vi "#241_MAV_MSG_VIBRATION_DECODE.vi"(11 "mavlink_payload":u8[](array[numeric])) -> (3 "VIBRATION":T1)   [LabVIEW 2023]
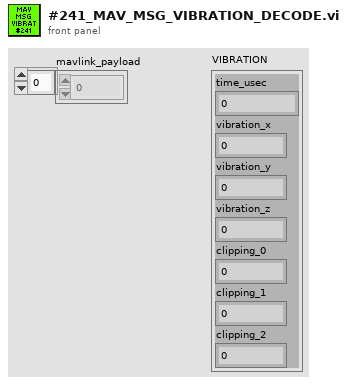
[diagram p1: front panel]
types:
  T1 = cluster{"time_usec":u64, "vibration_x":sgl, "vibration_y":sgl, "vibration_z":sgl, "clipping_0":u32, "clipping_1":u32, "clipping_2":u32}
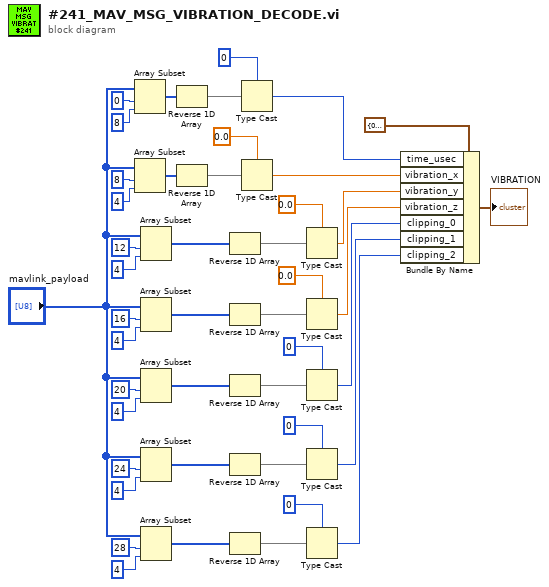
[diagram p0: block diagram]
diagram:
  n1 = Array Subset(array="mavlink_payload", index=0 ("Index"), length=8) -> (w42:u8[])
  n2 = Array Subset(array="mavlink_payload", index=8 ("Index"), length=4) -> (w36:u8[])
  n3 = Array Subset(array="mavlink_payload", index=12 ("Index"), length=4) -> (w30:u8[])
  n4 = Array Subset(array="mavlink_payload", index=16 ("Index"), length=4) -> (w24:u8[])
  n5 = Array Subset(array="mavlink_payload", index=20 ("Index"), length=4) -> (w18:u8[])
  n6 = Array Subset(array="mavlink_payload", index=24 ("Index"), length=4) -> (w12:u8[])
  n7 = Array Subset(array="mavlink_payload", index=28 ("Index"), length=4) -> (w6:u8[])
  n8 = Reverse 1D Array(array=w42) -> (reversed array=w41:u8[])
  n9 = Reverse 1D Array(array=w36) -> (reversed array=w35:u8[])
  n10 = Reverse 1D Array(array=w30) -> (reversed array=w29:u8[])
  n11 = Reverse 1D Array(array=w24) -> (reversed array=w23:u8[])
  n12 = Reverse 1D Array(array=w18) -> (reversed array=w17:u8[])
  n13 = Reverse 1D Array(array=w12) -> (reversed array=w11:u8[])
  n14 = Reverse 1D Array(array=w6) -> (reversed array=w5:u8[])
  n15 = Type Cast(type=u64 0 ("Index"), x=w41) -> (*(type *) &x=w38:u64)
  n16 = Type Cast(type=sgl 0.0 ("Index"), x=w35) -> (*(type *) &x=w32:sgl)
  n17 = Type Cast(type=sgl 0.0 ("Index"), x=w29) -> (*(type *) &x=w26:sgl)
  n18 = Type Cast(type=sgl 0.0 ("Index"), x=w23) -> (*(type *) &x=w20:sgl)
  n19 = Type Cast(type=u32 0 ("Index"), x=w17) -> (*(type *) &x=w14:u32)
  n20 = Type Cast(type=u32 0 ("Index"), x=w11) -> (*(type *) &x=w8:u32)
  n21 = Type Cast(type=u32 0 ("Index"), x=w5) -> (*(type *) &x=w1:u32)
  n22 = Bundle By Name(cluster=T1 {"time_usec"=0, "vibration_x"=0.0, "vibration_y"=0.0, "vibration_z"=0.0, "clipping_0"=0, "clipping_1"=0, "clipping_2"=0} ("VIBRATION"), "time_usec"=w38, "vibration_x"=w32, "vibration_y"=w26, "vibration_z"=w20, "clipping_0"=w14, "clipping_1"=w8, "clipping_2"=w1) -> (→"VIBRATION":T1)
